vi "Multiply Force.vi"(10 "force in":dbl, 11 "Flathead in":refnum<class "Flathead.lvclass">) -> (2 "force out":dbl)   [LabVIEW 2023, in "Flathead.lvclass"]
uses:
  Flathead.lvclass
panel:
  in  "broken message":string="Flathead screwdriver breaks when too much force is applied. This is why woodworkers get upset when people use their screwdrivers as levers.\nForce = %f"
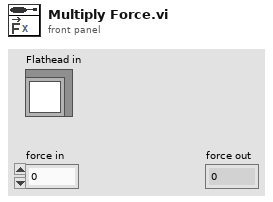
[diagram p1: front panel]
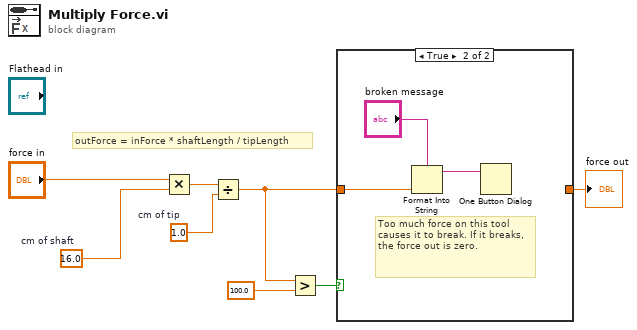
[diagram p0: block diagram]
diagram:
  w6 = 16.0  # cm of shaft
  w7 = 1.0  # cm of tip
  # "outForce = inForce * shaftLength / tipLength"
  n1 = Multiply(x="force in", y=w6) -> (x*y=w8:dbl)
  n2 = Divide(x=w8, y=w7) -> (x/y=w1:dbl)
  n3 = Greater?(x=w1, y=100.0) -> (0:w4:bool)
  n4 = case shown="True" w4 {
    tunnel: [w9 _] -> w2
    tunnel: w1 -> [w9 w11]
    frame False {
    }
    frame True {
      # "Too much force on this tool causes it to break. If it breaks, the force out is zero."
      n5 = Format Into String(format string="broken message", w11) -> (resulting string=w10:string)  [unwired: 2 in, 1 out]
      n6 = One Button Dialog(message=w10) -> ()  [unwired: 1 in, 1 out]
    }
  }
  "force out" <- w2
